vi "PSTR-Insert Data.vi"(0 "Data in":T1, 2 "Finished":bool, 5 "iLevel":i32, 7 "PSD":dbl[][](array[numeric]), 9 "PSTR":dbl[](array[numeric]), 11 "Spont":bool, 12 "Amplitude":dbl) -> (4 "Data out":T1)   [LabVIEW 2020]
uses:
  Typedefs/PSTR-Data.ctl
  Typedefs/PSTR-Model Fit.ctl
  Typedefs/PSTR-Fit Parameters.ctl
  26ba39a7-6fd3-4b4a-a27a-3f538fda82a7.vi
  e71cbe04-6c73-421f-b8cd-2fd49273d928.vi
panel:
  # "NF x NL x 2 x Npts"
  # "NF x NL x Npts"
  # "NF x NL"
  # "NF x NL x 2 x Npts"
  # "NF x NL x Npts"
  # "NF x NL"
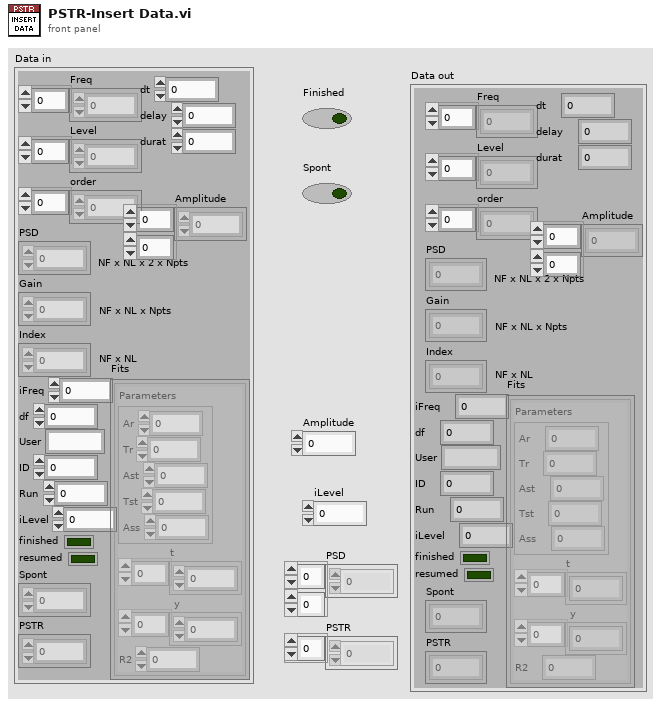
[diagram p1: front panel]
types:
  T1 = typedef "PSTR-Data.ctl" = cluster{"Freq":dbl[], "Level":dbl[], "order":i32[], "PSD":dbl[][][][], "Gain":dbl[][][], "Index":dbl[][], "iFreq":i32, "df":dbl, "User":string, "ID":i32, "Run":i32, "iLevel":i32, "finished":bool, "resumed":bool, "Spont":dbl[][], "PSTR":dbl[][][], "dt":dbl, "delay":dbl, "durat":dbl, "Fits":T2[][], "Amplitude":dbl[][]}
  T2 = typedef "PSTR-Model Fit.ctl" = cluster{"Parameters":T3, "t":dbl[], "y":dbl[], "R2":dbl}
  T3 = typedef "PSTR-Fit Parameters.ctl" = cluster{"Ar":dbl, "Tr":dbl, "Ast":dbl, "Tst":dbl, "Ass":dbl}
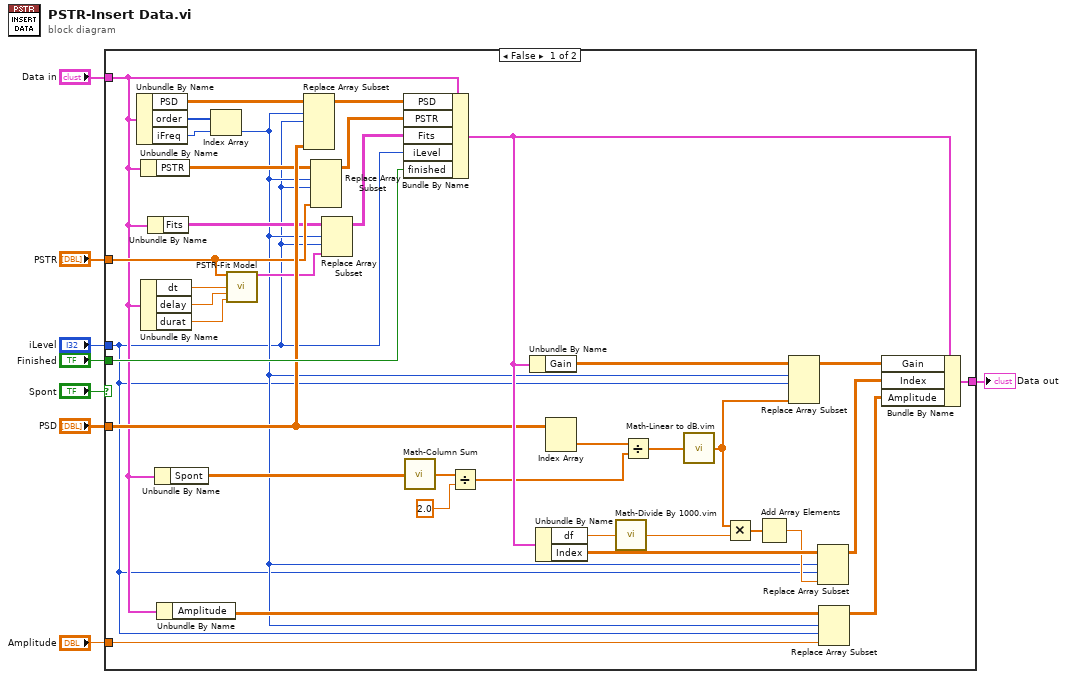
[diagram p0: block diagram]
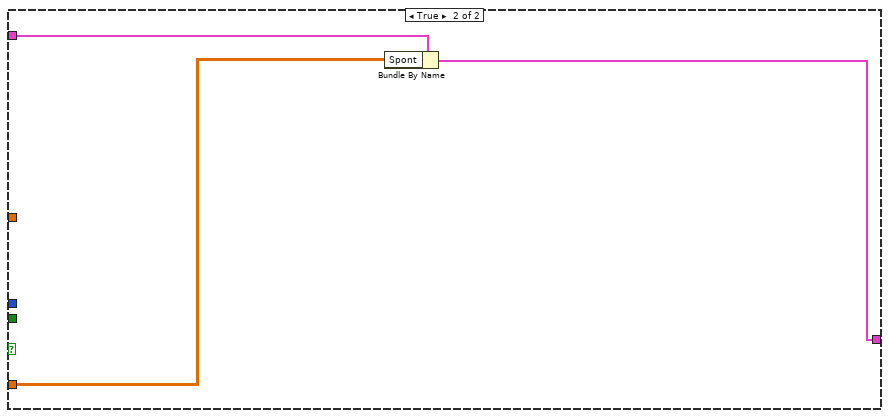
[diagram p2: hidden frame]
diagram:
  n1 = case shown="False" "Spont" {
    tunnel: "Data in" -> [w14 w48]
    tunnel: [w44 w49] -> w7
    tunnel: "iLevel" -> [w10 _]
    tunnel: "Finished" -> [w43 _]
    tunnel: "PSD" -> [w27 w47]
    tunnel: "PSTR" -> [w23 _]
    tunnel: "Amplitude" -> [w9 _]
    frame False {
      n2 = Unbundle By Name(w14) -> ("PSD"=w46:dbl[][][][], "order"=w21:i32[], "iFreq"=w20:i32)
      n3 = Unbundle By Name(w14) -> ("PSTR"=w25:dbl[][][])
      n4 = Unbundle By Name(w14) -> ("dt"=w22:dbl, "delay"=w15:dbl, "durat"=w16:dbl)
      n5 = Unbundle By Name(w14) -> ("Fits"=w19:T2[][])
      n6 = Unbundle By Name(w14) -> ("Spont"=w31:dbl[][])
      n7 = Unbundle By Name(w14) -> ("Amplitude"=w13:dbl[][])
      n8 = Index Array(array=w21, index=w20) -> (element=w11:i32)
      n9 = call "PSTR-Fit Model.vi"("PSTH"=w23, "dt (ms)"=w22, "delay (ms)"=w15, "durat (ms)"=w16) -> ("Fit"=w17:T2)  [unwired: 11 in]
      n10 = Replace Array Subset(array=w46, new element=w27, index (dim 0)=w11, index (dim 1)=w10) -> (w42:dbl[][][][])  [unwired: 2 in]
      n11 = Replace Array Subset(array=w25, new element=w23, index (dim 0)=w11, index (dim 1)=w10) -> (w24:dbl[][][])  [unwired: 1 in]
      n12 = Replace Array Subset(array=w19, new element=w17, index (row)=w11, index (col)=w10) -> (w18:T2[][])
      n13 = Bundle By Name(cluster=w14, "PSD"=w42, "PSTR"=w24, "Fits"=w18, "iLevel"=w10, "finished"=w43) -> (w45:T1)
      n14 = call "Math-Column Sum.vi"("2D Array"=w31) -> ("Column sums"=w30:dbl[])
      n15 = Divide(x=w30, y=2.0) -> (x/y=w28:dbl[])
      n16 = Unbundle By Name(w45) -> ("Gain"=w40:dbl[][][])
      n17 = Unbundle By Name(w45) -> ("df"=w34:dbl, "Index"=w36:dbl[][])
      n18 = Index Array(array=w27) -> (element=w41:dbl[])  [unwired: 2 in]
      n19 = call "Math-Divide By 1000.vim"("X"=w34) -> ("1000X"=w32:dbl)
      n20 = Divide(x=w41, y=w28) -> (x/y=w38:dbl[])
      n21 = call "Math-Linear to dB.vim"("linear"=w38) -> ("dB"=w33:dbl[])
      n22 = Multiply(x=w33, y=w32) -> (x*y=w37:dbl[])
      n23 = Add Array Elements(numeric array=w37) -> (sum=w26:dbl)
      n24 = Replace Array Subset(array=w40, new element=w33, index (dim 0)=w11, index (dim 1)=w10) -> (w39:dbl[][][])  [unwired: 1 in]
      n25 = Replace Array Subset(array=w36, new element=w26, index (row)=w11, index (col)=w10) -> (w35:dbl[][])
      n26 = Replace Array Subset(array=w13, new element=w9, index (row)=w11, index (col)=w10) -> (w12:dbl[][])
      n27 = Bundle By Name(cluster=w45, "Gain"=w39, "Index"=w35, "Amplitude"=w12) -> (w44:T1)
    }
    frame True {
      n28 = Bundle By Name(cluster=w48, "Spont"=w47) -> (w49:T1)
    }
  }
  "Data out" <- w7
